vi "Do.vi"(8 "error in (no error)":errorcluster, 10 "Actor in":refnum<class "Actor.lvclass">, 11 "Store Data Msg":refnum<class "Store Data Msg.lvclass">) -> (0 "error out":errorcluster, 2 "Actor out":refnum<class "Actor.lvclass">)   [LabVIEW 2014, in "Store Data Msg.lvclass"]
doc: "This VI delivers the message to the actor by calling the appropriate method(s) on the actor."
uses:
  Store Data Msg.lvclass
  <vilib>/ActorFramework/Actor/Actor.lvclass
  StorageService.lvclass
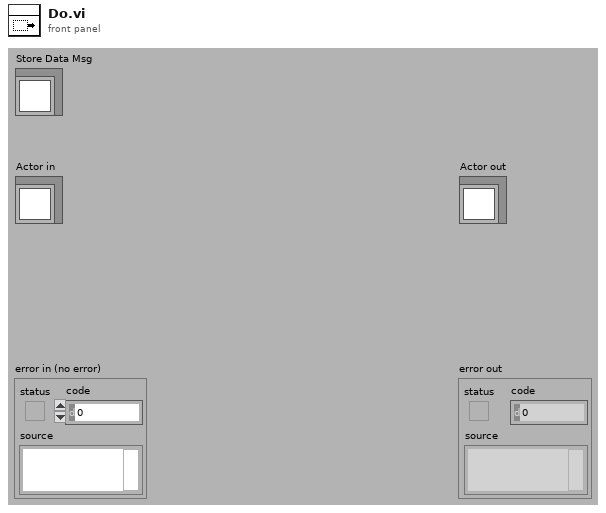
[diagram p1: front panel]
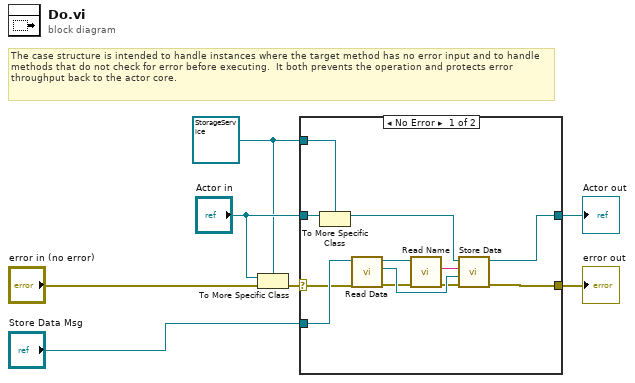
[diagram p0: block diagram]
diagram:
  w2 = refnum<class "StorageService.lvclass"> refnum ("Actor in")
  # "The case structure is intended to handle instances where the target method has no error input and to handle methods that do not check for error before executing.  It both prevents the operation and protects error throughput back to the actor core."
  n1 = To More Specific Class(target class=w2, reference="Actor in", error in="error in (no error)") -> (error out=w6:errorcluster)  [unwired: 1 out]
  n2 = case shown="No Error" w6 {
    selector: w6 -> [w8 w21]
    tunnel: [w19 w21] -> w5
    tunnel: [w18 w20] -> w4
    tunnel: "Actor in" -> [w17 w20]
    tunnel: w2 -> [w16 _]
    tunnel: "Store Data Msg" -> [w14 _]
    frame No Error {
      n3 = To More Specific Class(target class=w16, reference=w17) -> (specific class reference=w15:refnum<class "StorageService.lvclass">)  [unwired: 1 in, 1 out]
      n4 = call-dynamic "Read Data.vi"("error in (no error)"=w8, "Data Msg in"=w14) -> ("error out"=w10:errorcluster, "AbstractData.lvclass"=w13:refnum<class "AbstractData.lvclass">, "Data Msg out"=w9:refnum<class "Store Data Msg.lvclass">)  [unwired: 7 in]
      n5 = call-dynamic "Read Name.vi"("error in (no error)"=w10, "Data Msg in"=w9) -> ("error out"=w11:errorcluster, "Name"=w12:string)  [unwired: 7 in, 1 out]
      n6 = call "Store Data.vi"("error in (no error)"=w11, "Data"=w13, "Name"=w12, "StorageService in"=w15) -> ("error out"=w19:errorcluster, "StorageService out"=w18:refnum<class "StorageService.lvclass">)  [unwired: 6 in]
    }
    frame Error {
      # "If type check fails, pass the original object out again."
    }
  }
  "error out" <- w5
  "Actor out" <- w4
